vi "Data FG.vi"(7 "Data Action":T1, 8 "error in (no error)":errorcluster, 11 "Data In":refnum<class "Rename.lvclass">) -> (0 "error out":errorcluster, 3 "Data Out":refnum<class "Rename.lvclass">)   [LabVIEW 2015, in "Generic Module Library.lvlib" / "Template G_Module.lvlib"]
uses:
  Template G_Module.lvlib
  Module Class/Rename.lvclass
  Data Actions.ctl
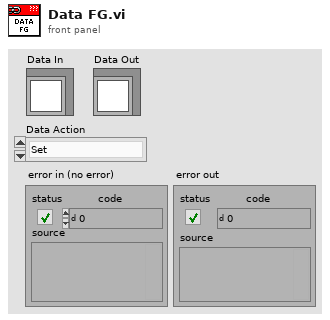
[diagram p1: front panel]
types:
  T1 = typedef "Generic Module Library.lvlib/Template G_Module.lvlib/Data Actions.ctl" = enum16{"Set", "Get"}
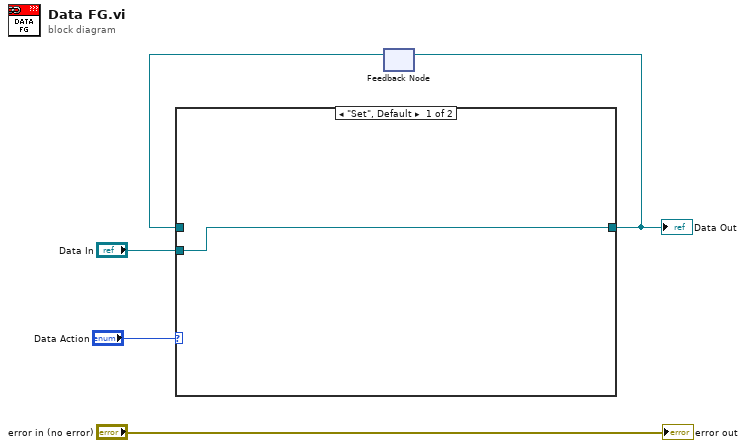
[diagram p0: block diagram]
diagram:
  n1 = feedback #1() -> (w4:refnum<class "Rename.lvclass">)  [unwired: 1 in]
  n2 = case shown="\"Set\", Default" "Data Action" {
    tunnel: "Data In" -> [w6 _]
    tunnel: [w6 w7] -> w5
    tunnel: w4 -> [_ w7]
    frame "Set", Default {
    }
    frame "Get" {
    }
  }
  "Data Out" <- w5
  n3 = feedback-in #1(w5) -> ()
  "error out" <- "error in (no error)"
